vi "Get DBL from User.vi"(4 "number format":T1, 6 "digits(2)":u8=2, 8 "error in":errorcluster, 9 "timeout (s)":dbl=300.0, 10 "default value(0)":dbl, 11 "prompt":string) -> (0 "error out":errorcluster, 1 "timeout?":bool, 2 "cancelled?":bool, 3 "DBL out":dbl)   [LabVIEW 2010]
uses:
  type defs/number formats.ctl
panel:
  out "prompt display":string
  in  "user input":dbl format="%.2f"
  in  "cancel btn":bool
  in  "OK btn":bool
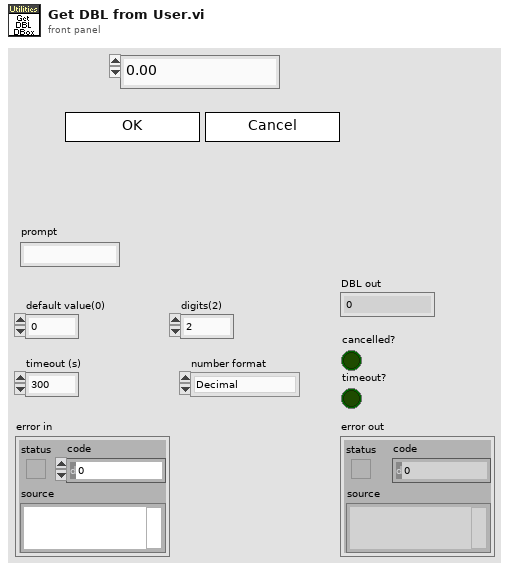
[diagram p1: front panel]
types:
  T1 = typedef "number formats.ctl" = enum16{"Decimal", "Scientific", "Engineering", "Binary", "Octal", "Hexadecimal", "Relative Time", "Time and Date", "SI", "Custom"}
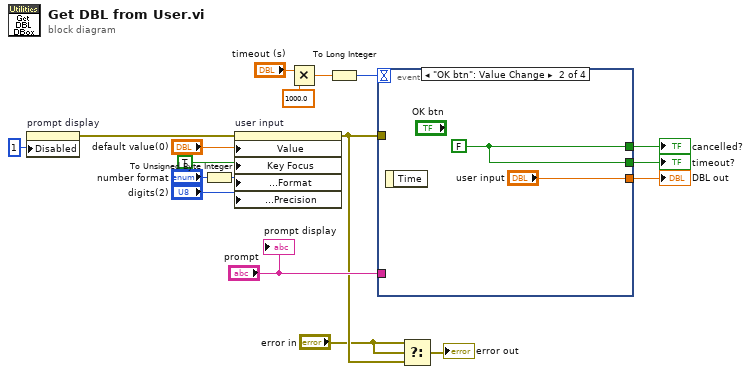
[diagram p0: block diagram]
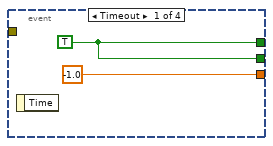
[diagram p2: hidden frame]
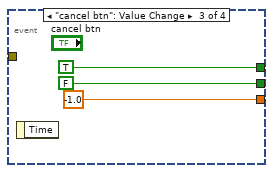
[diagram p3: hidden frame]
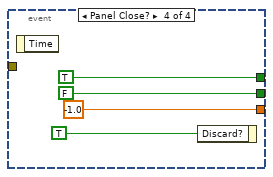
[diagram p4: hidden frame]
diagram:
  n1 = property on="prompt display" class="Str"("Disabled"=u8 1) -> (error out=w2:errorcluster)  [unwired: 2 in, 1 out]
  n2 = To Unsigned Byte Integer(number="number format") -> (unsigned 8bit integer=w6:u8)
  n3 = property on="user input" class="DigNum (strict)"(error in=w2, "Value"="default value(0)", "Key Focus"=TRUE, "Numeric Text.Display Format:Format"=w6, "Numeric Text.Display Format:Precision"="digits(2)") -> (error out=w5:errorcluster)  [unwired: 1 in, 1 out]
  n4 = Multiply(x="timeout (s)", y=1000.0) -> (x*y=w15:dbl)
  n5 = To Long Integer(number=w15) -> (32bit integer=w16:i32)
  n6 = event shown="[1] \"OK btn\": Value Change" {
    selector: _ -> [_ _ _ _]
    dyn-events: _ -> [_ _ _ _]
    timeout: w16 -> [_ _ _ _]
    tunnel: w5 -> [_ _ _ _]
    tunnel: "prompt" -> [_ _ _ _]
    tunnel: [w20 w22 TRUE TRUE] -> w11
    tunnel: [w20 w22 FALSE FALSE] -> w10
    tunnel: [-1.0 ("user input") "user input" -1.0 ("user input") -1.0 ("user input")] -> w9
    event Timeout {
      w20 = TRUE
      n7 = event-data() -> ()  [unwired: 2 out]
    }
    event "OK btn": Value Change {
      w22 = FALSE
      n8 = event-data() -> ()  [unwired: 2 out]
    }
    event "cancel btn": Value Change {
      n9 = event-data() -> ()  [unwired: 2 out]
    }
    event Panel Close? {
      n10 = event-data() -> ()  [unwired: 2 out]
      n11 = event-data("Discard?"=TRUE) -> ()  [unwired: 1 in, 1 out]
    }
  }
  "DBL out" <- w9
  "cancelled?" <- w11
  "timeout?" <- w10
  n12 = Select(t="error in", s="error in", f=w5) -> (s? t:f=→"error out":errorcluster)
  "prompt display" <- "prompt"
